vi "T7MOD_Write_UINT32_Registers.vi"(7 "UINT32 to Write":u32[](array[numeric]), 8 "error in":errorcluster, 9 "Starting Address":i32=55120, 10 "Remote Port":u16=502, 11 "Remote IP Address":string="192.168.1.15") -> (0 "error out":errorcluster, 1 "Written At":timestamp)   [LabVIEW 2015]
uses:
  Serial Link Layer/NI_Modbus_Cleaned/NI Modbus121Clean.llb/MB Ethernet Master Query Write Multiple Registers (poly).vi
panel:
  # "Input"
  # "TCP Parameters"
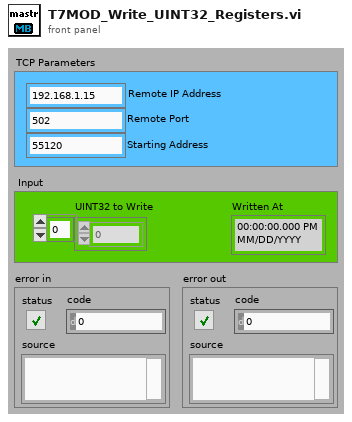
[diagram p1: front panel]
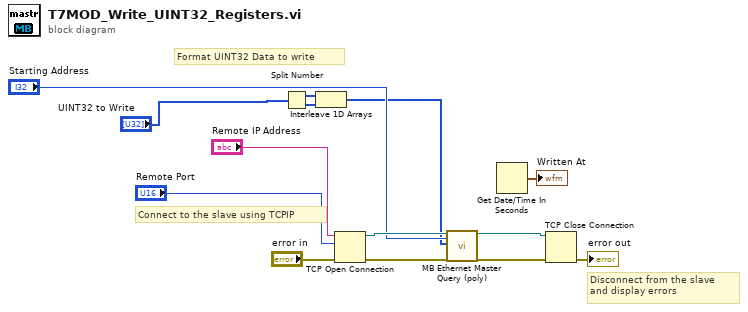
[diagram p0: block diagram]
diagram:
  # "Format UINT32 Data to write"
  # "Disconnect from the slave\nand display errors"
  # "Connect to the slave using TCPIP"
  n1 = Split Number(x="UINT32 to Write") -> (hi(x)=w3:u16[], lo(x)=w2:u16[])
  n2 = Interleave 1D Arrays(w3, w2) -> (w1:u16[])
  n3 = TCP Open Connection(address="Remote IP Address", remote port or service name="Remote Port", error in (no error)="error in") -> (connection ID=w12:refnum<k5>, error out=w11:errorcluster)  [unwired: 2 in]
  n4 = call-poly "MB Ethernet Master Query (poly).vi"("TCP Connection Refnum in"=w12, "Starting Address"="Starting Address", "Registers"=w1, "error in"=w11) -> ("TCP Connection Refnum (dup)"=w9:refnum<k5>, "error out"=w10:errorcluster)  [unwired: 13 in, 1 out]
  n5 = Get Date/Time In Seconds() -> (seconds since 1Jan1904=→"Written At":timestamp)
  n6 = TCP Close Connection(connection ID=w9, error in (no error)=w10) -> (error out=→"error out":errorcluster)  [unwired: 2 out]
